vi "NGread_imp.vi"(0 "Unresolved URL":string, 1 "buffer value limit":u32=1, 5 "Cached URL":string, 7 "GetTimestamp":bool, 9 "buffer size limit":u32=4294967295, 11 "error in":errorcluster, 12 "Type":variant) -> (4 "Data":variant, 10 "time":timestamp, 15 "error out":errorcluster)   [LabVIEW 2020]
uses:
  nitaglv.dll
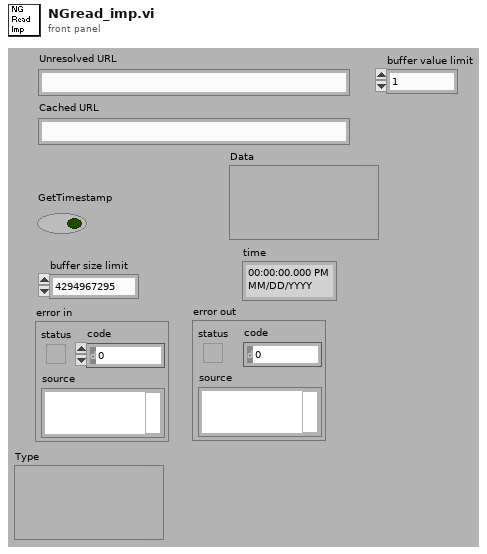
[diagram p1: front panel]
types:
  T1 = cluster{"timestamp":bool, "write":bool, "buffer size limit":u32, "buffer value limit":u32, "delta filter":bool}
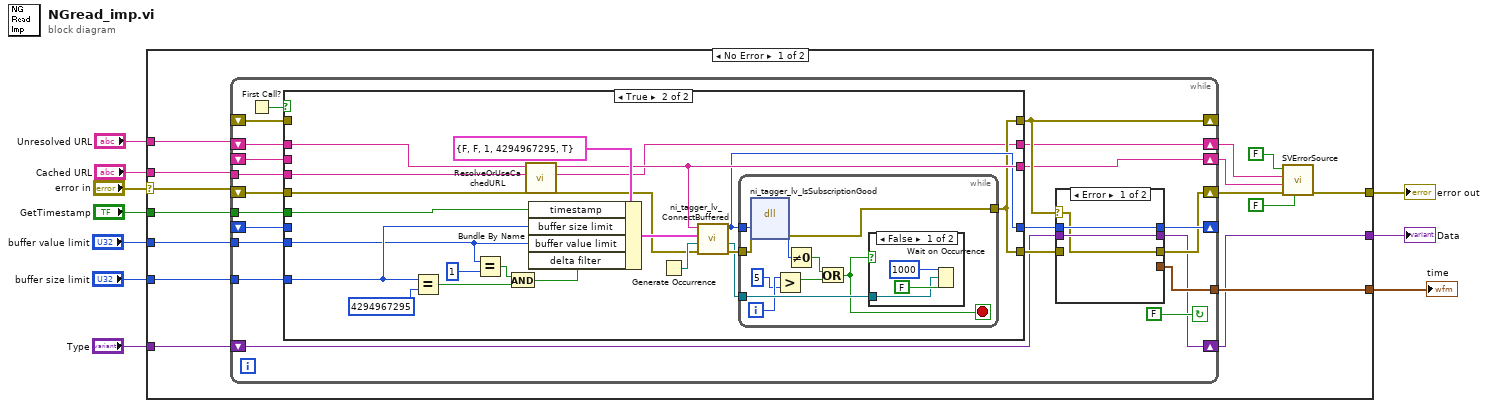
[diagram p0: block diagram]
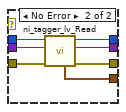
[diagram p2: hidden frame]
diagram:
  n1 = case shown="No Error" "error in" {
    selector: "error in" -> [w25 w97]
    tunnel: [w17 w97] -> w9
    tunnel: [w24 _] -> w1
    tunnel: [w23 w96] -> w8
    tunnel: "GetTimestamp" -> [w22 _]
    tunnel: "Unresolved URL" -> [w13 _]
    tunnel: "buffer size limit" -> [w21 _]
    tunnel: "buffer value limit" -> [w20 _]
    tunnel: "Type" -> [w19 w96]
    tunnel: "Cached URL" -> [w15 _]
    frame No Error {
      n2 = while {
        shift-right: [w42] -> _
        shift-left: _ -> [w43]
        tunnel: [w38] -> w24
        tunnel: w22 -> [w36]
        tunnel: w21 -> [w35]
        tunnel: w20 -> [w34]
        tunnel: w15 -> [w32]
        shift-right: [w37] -> w23
        shift-left: w19 -> [w33]
        shift-right: [w39] -> w18
        shift-left: w25 -> [w40]
        shift-right: [w27] -> w12
        shift-left: w13 -> [w45]
        shift-right: [w29] -> _
        shift-left: _ -> [w31]
        shift-right: [w26] -> w11
        shift-left: _ -> [w28]
        stop <- FALSE continue-if-true
        n3 = First Call?() -> (First Call?: T/F=w41:bool)
        n4 = case shown="True" w41 {
          tunnel: w45 -> [w57 w74]
          tunnel: [w61 w64] -> w30
          tunnel: [w60 w63] -> w44
          tunnel: w43 -> [w61 _]
          tunnel: w40 -> [w60 w73]
          tunnel: w36 -> [_ w71]
          tunnel: w35 -> [_ w70]
          tunnel: w34 -> [_ w69]
          tunnel: w32 -> [_ w68]
          tunnel: [w58 w67] -> w26
          tunnel: [w59 w63] -> w29
          tunnel: w31 -> [w59 _]
          tunnel: w28 -> [w58 _]
          tunnel: [w57 w62] -> w27
          frame False {
          }
          frame True {
            n5 = Equal?(x=w70, y=u32 4294967295 ("buffer value limit")) -> (x = y?=w77:bool)
            n6 = Equal?(x=w69, y=u32 1) -> (x = y?=w76:bool)
            n7 = And(x=w76, y=w77) -> (x .and. y?=w75:bool)
            n8 = call <vilib>:"ResolveOrUseCachedURL.vi"("error in (no error)"=w73, "Cached Resolved URL"=w68, "Unresolved URL"=w74) -> ("error out"=w72:errorcluster, "Unresolved URL out"=w62:string, "Resolved URL out"=w67:string)  [unwired: 6 in]
            n9 = Bundle By Name(cluster=T1 {"timestamp"=FALSE, "write"=FALSE, "buffer size limit"=1, "buffer value limit"=4294967295, "delta filter"=TRUE} ("options"), "timestamp"=w71, "buffer size limit"=w70, "buffer value limit"=w69, "delta filter"=w75) -> (w80:T1)
            n10 = Generate Occurrence() -> (w82:refnum<k4>)
            n11 = call <vilib>:"ni_tagger_lv_ConnectBuffered.vi"("error in (no error)"=w72, "read in"=w82, "options"=w80, "path"=w67) -> ("error out"=w66:errorcluster, "read out"=w65:refnum<k4>, "item"=w64:u32)  [unwired: 1 in]
            n12 = while {
              tunnel: w64 -> [w91]
              tunnel: w65 -> [w92]
              tunnel: [w89] -> w63
              tunnel: w66 -> [w88]
              i -> [w87]
              stop <- w83 stop-if-true
              n13 = dll-call lib="nitaglv.*" fn="ni_tagger_lv_IsSubscriptionGood" label="IsSubscriptionGood"("itemRefnum"=w91, "error out"=w88) -> (w90:i32, "error out"=w89:errorcluster)  [unwired: 4 in, 2 out]
              n14 = Greater?(x=w87, y=5 ("x")) -> (0:w85:bool)
              n15 = Not Equal To 0?(x=w90) -> (x != 0?=w84:bool)
              n16 = Or(x=w84, y=w85) -> (x .or. y?=w83:bool)
              n17 = case shown="False" w83 {
                tunnel: w92 -> [w93 _]
                frame False {
                  n18 = Wait on Occurrence(1:FALSE ("ignore previous (T)"), 2:w93, 3:1000 ("ms timeout (-1)")) -> ()  [unwired: 1 out]
                }
                frame True {
                }
              }
            }
          }
        }
        n19 = case shown="Error" w29 {
          selector: w29 -> [w47 _]
          tunnel: w44 -> [_ w56]
          tunnel: [w48 w55] -> w42
          tunnel: [w47 w54] -> w39
          tunnel: [_ w53] -> w38
          tunnel: [w49 w52] -> w37
          tunnel: w33 -> [w49 w51]
          tunnel: w30 -> [w48 w50]
          frame Error {
          }
          frame No Error {
            n20 = call <vilib>:"ni_tagger_lv_Read.vi"("error in"=w56, "Type"=w51, "item in"=w50) -> ("error out"=w54:errorcluster, "value"=w52:variant, "item out"=w55:u32, "time"=w53:timestamp)  [unwired: 4 in, 1 out]
          }
        }
      }
      n21 = call <vilib>:"SVErrorSource.vi"("RT?"=FALSE, "error in"=w18, "Resolved URL"=w11, "Unresolved URL"=w12, "Write?"=FALSE) -> ("error out"=w17:errorcluster)  [unwired: 6 in]
    }
    frame Error {
    }
  }
  "error out" <- w9
  "Data" <- w8
  "time" <- w1
